vi "Colour Items of a JSON string control.vi"(7 "Maximum UI Property calls":i32=-1, 10 "String Control":refnum<vi>, 11 "JSON":string) -> ()   [LabVIEW 2017, in "JSONtext.lvlib"]
doc: "Writes the input JSON to a string control and colour the elements for better readability. Note that this may be slow for large JSON structures. You may set a limit to number of elements that are actually coloured in order to ensure the VI completes in a reasonable amount of time (the default of -1 means no limit)."
uses:
  JSONtext.lvlib
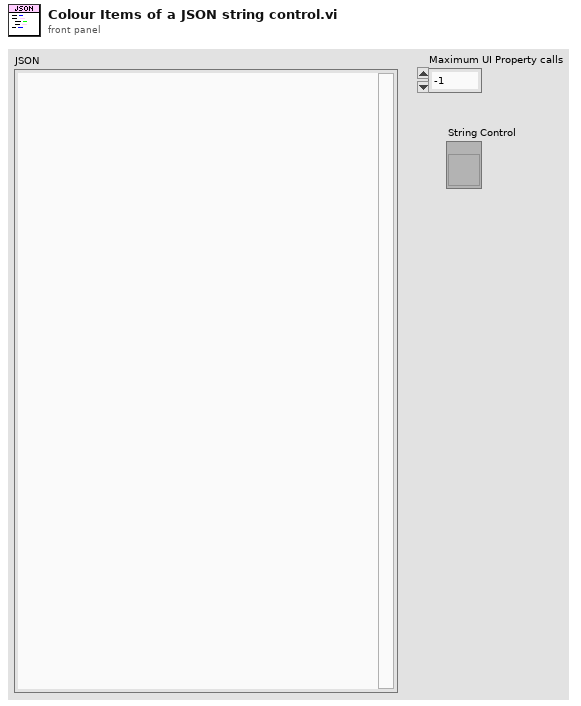
[diagram p1: front panel]
types:
  T1 = typedef "JSONtext.lvlib/JSON Value Type.ctl" = enum16{"Not a JSON Value", "JSON Object", "JSON Array", "String", "Number", "true", "false", "null"}
  T2 = cluster{"Value start out":i32, "Offset past match":i32, "JSON Value Type":T1}[]
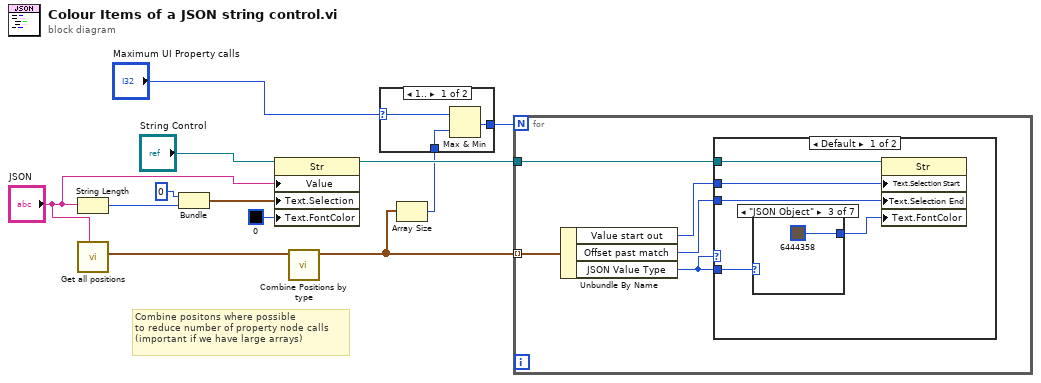
[diagram p0: block diagram]
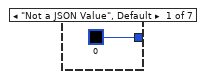
[diagram p3: hidden frame]
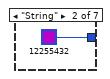
[diagram p4: hidden frame]
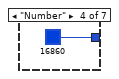
[diagram p5: hidden frame]
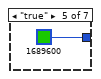
[diagram p6: hidden frame]
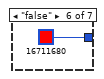
[diagram p7: hidden frame]
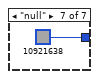
[diagram p8: hidden frame]
diagram:
  # "Combine positons where possible \nto reduce number of property node calls\n(important if we have large arrays)"
  n1 = String Length(string="JSON") -> (length=w11:i32)
  n2 = call "Get all positions.vi"("JSON"="JSON") -> ("Array"=w5:T2)  [unwired: 8 in, 2 out]
  n3 = Bundle("Selection Start"=u32 0, w11) -> (w10:cluster{"Selection Start":u32, i32})  [unwired: 1 in]
  n4 = property on="Property Node" class="Str"(reference="String Control", "Value"="JSON", "Text.Selection"=w10, "Text.FontColor"=u32 0) -> (reference out=w8:refnum<vi>)  [unwired: 1 in, 1 out]
  n5 = call "Combine Positions by type.vi"("Array in"=w5) -> ("Array out"=w2:T2)  [unwired: 10 in]
  n6 = Array Size(array=w2) -> (size(s)=w1:i32)
  n7 = case shown="1.." "Maximum UI Property calls" {
    selector: "Maximum UI Property calls" -> [w13 _]
    tunnel: [w15 w16] -> w4
    tunnel: w1 -> [w14 w16]
    frame 1.. {
      n8 = Max & Min(x=w13, y=w14) -> (min(x,y)=w15:i32)  [unwired: 1 out]
    }
    frame ..0 {
    }
  }
  n9 = for {
    N: w4 -> [_]
    tunnel: w2 -> [w21] mode=indexing
    tunnel: w8 -> [w17]
    n10 = Unbundle By Name(w21) -> ("Value start out"=w20:i32, "Offset past match"=w19:i32, "JSON Value Type"=w18:T1)
    n11 = case shown="Default" w18 {
      tunnel: w18 -> [w26 _]
      tunnel: w20 -> [w24 _]
      tunnel: w19 -> [w23 _]
      tunnel: w17 -> [w22 _]
      frame Default {
        n12 = case shown="\"JSON Object\"" w26 {
          tunnel: [u32 0 u32 12255432 u32 6444358 u32 16860 u32 1689600 u32 16711680 u32 10921638] -> w25
          frame "Not a JSON Value", Default {
          }
          frame "String" {
          }
          frame "JSON Object" {
          }
          frame "Number" {
          }
          frame "true" {
          }
          frame "false" {
          }
          frame "null" {
          }
        }
        n13 = property on="Property Node" class="Str"(reference=w22, "Text.Selection Start"=w24, "Text.Selection End"=w23, "Text.FontColor"=w25) -> ()  [unwired: 1 in, 2 out]
      }
      frame "JSON Object" {
      }
    }
  }
